vi "CreateHDF5NoDig.vi"() -> (0 "error out":errorcluster, 3 "File Handle":T1=16777216 format="%.0x")   [LabVIEW 2014]
uses:
  <vilib>/addons/h5labview2/base/hid_t.ctl
panel:
  in  "Material in Tank":string(combo)
  in  "Optional Comments":string
  in  "Run Type":string(combo)
  in  "Click OK when all data are entered.":bool
  in  "QDC Info, Ch0 - 7, left to right":T2={"Chanel Description"=["H0", "H1", "H2", "H3", "H4", "H5"], "Only Hodo?"=[TRUE, TRUE, TRUE, TRUE, TRUE, TRUE]}
  in  "Scaler Info":T2={"Chanel Description"=["H0", "H1", "H2", "H3", "H4", "H5", "CT", "M", "LED", "CT+M+LED", "S0", "S1", "S2", "S3", "S4", "S5", "S6", "S7"], "Only Hodo?"=[TRUE, TRUE, TRUE, TRUE, TRUE, TRUE, TRUE, TRUE, FALSE, FALSE, FALSE, FALSE, FALSE, FALSE, FALSE, FALSE, FALSE, FALSE]}
  in  "TDC Info":T2={"Chanel Description"=["H0", "H1", "H2", "H3", "H4", "H5", "CT", "M", "LED", "CT+M+LED", "S0", "S1", "S2", "S3", "S4", "S5", "S6", "S7"], "Only Hodo?"=[TRUE, TRUE, TRUE, TRUE, TRUE, TRUE, TRUE, FALSE, FALSE, FALSE, FALSE, FALSE, FALSE, FALSE, FALSE, FALSE, FALSE, FALSE]}
  in  "Trigger Bit Descriptions":string[](array[string])=["Cosmic Trigger (H0+H2)x(H1+H3)", "Multiplicity (S>1)", "LED pulse", "CT+M+LED"]
  in  "Thermocouple Location":string[](array[string])=["None", "None"]
  in  "HDF5 File Path":path=path "C:/Users/lbignell/Desktop/dummy3.h5" caption="HDF5 File Path (file name automatically generated)"
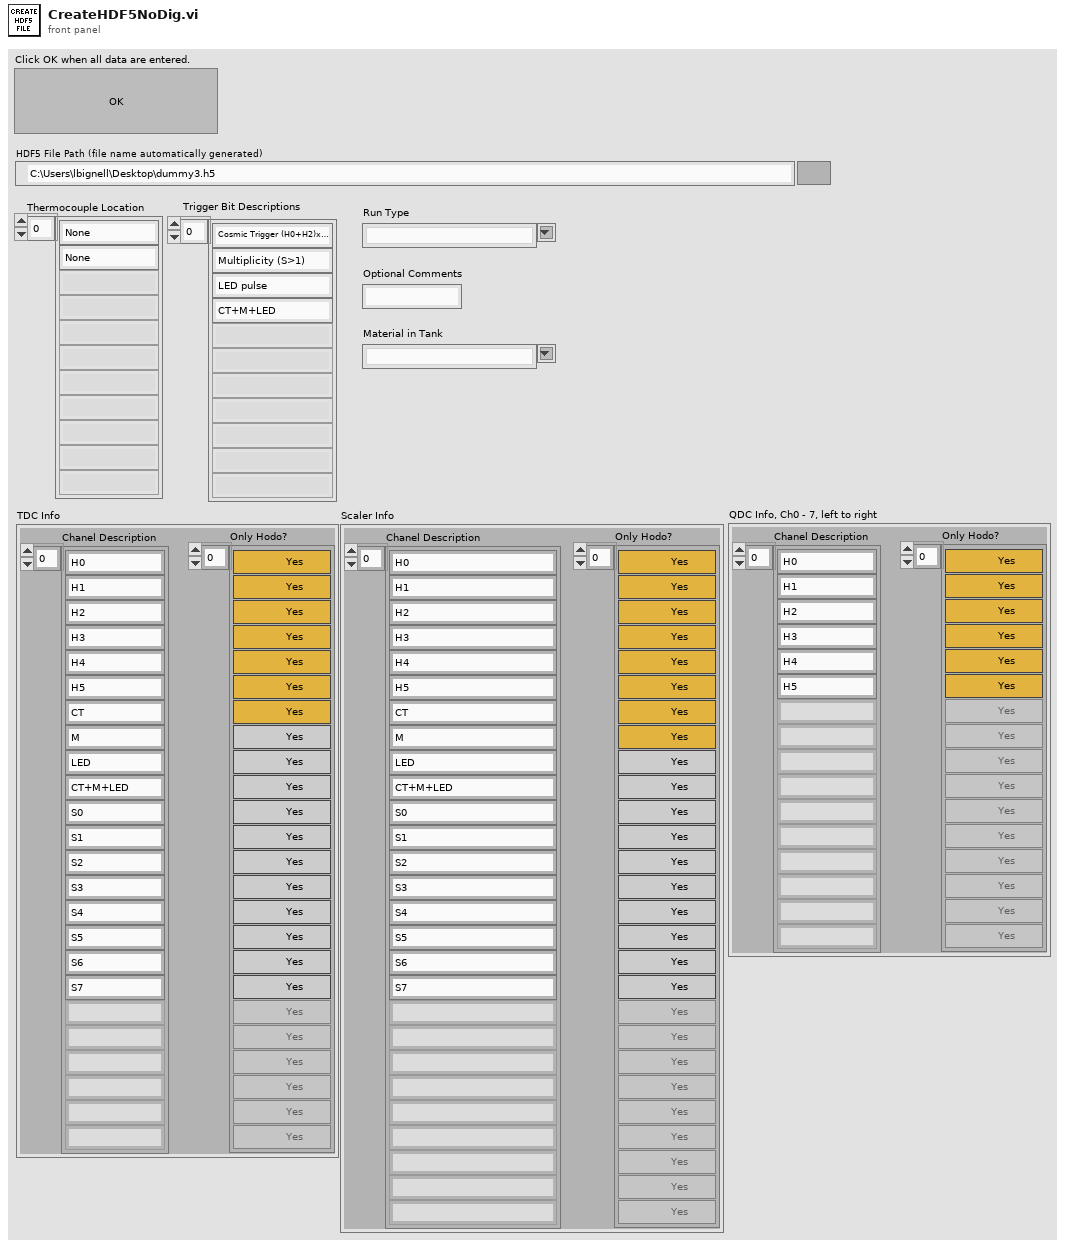
[diagram p1: front panel]
types:
  T1 = typedef "hid_t.ctl" = i32
  T2 = cluster{"Chanel Description":string[], "Only Hodo?":bool[]}
  T3 = cluster{"Module Description":string[], "Module Model":string[], "Module Address":u32[]}
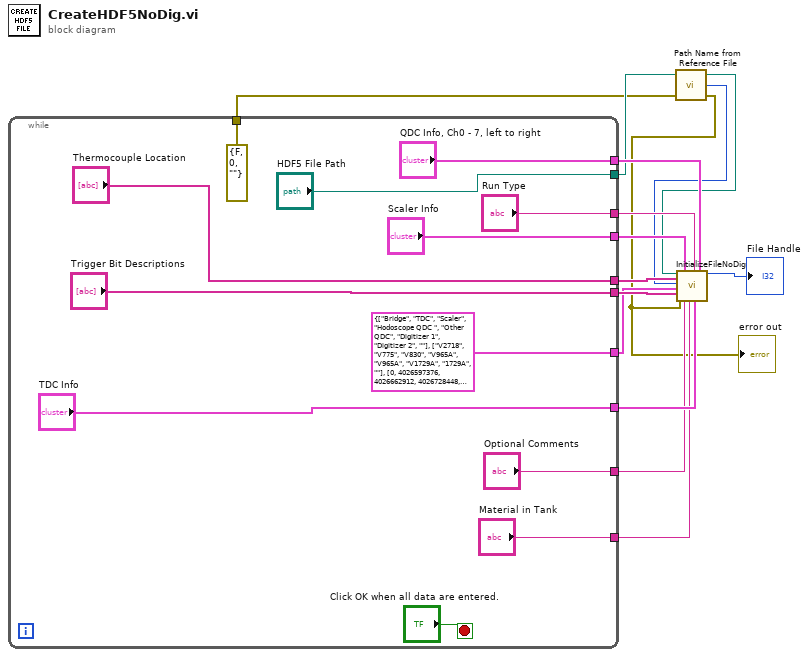
[diagram p0: block diagram]
diagram:
  n1 = while {
    tunnel: ["Thermocouple Location"] -> w15
    tunnel: ["Trigger Bit Descriptions"] -> w14
    tunnel: ["QDC Info, Ch0 - 7, left to right"] -> w13
    tunnel: ["Scaler Info"] -> w12
    tunnel: ["TDC Info"] -> w11
    tunnel: [T3 {"Module Description"=["Bridge", "TDC", "Scaler", "Hodoscope QDC ", "Other QDC", "Digitizer 1", "Digitizer 2", ""], "Module Model"=["V2718", "V775", "V830", "V965A", "V965A", "V1729A", "1729A", ""], "Module Address"=[0, 4026597376, 4026662912, 4026728448, 4026793984, 4026859520, 4026925056]} ("VME Configuration")] -> w9
    tunnel: ["Run Type"] -> w6
    tunnel: ["Optional Comments"] -> w7
    tunnel: ["Material in Tank"] -> w8
    tunnel: ["HDF5 File Path"] -> w5
    tunnel: [errorcluster {"status"=FALSE, "code"=0, "source"=""} ("error in")] -> w4
    stop <- "Click OK when all data are entered." stop-if-true
  }
  n2 = call "Path Name from Reference File"("error in"=w4, "Base Path"=w5) -> ("error out"=w3:errorcluster, "Run Number"=w2:i32, "Unique Path"=w1:path)  [unwired: 1 in]
  "error out" <- w3
  n3 = call "InitializeFileNoDig.vi"("File Path"=w1, "Thermocouple Location"=w15, "Run Number"=w2, "VME Configuration"=w9, "Trigger Bit Descriptions"=w14, "error in"=w3, "Scaler Info"=w12, "Optional Comments"=w7, "Material in Tank"=w8, "Run Type"=w6, "TDC Info"=w11, "QDC Info"=w13) -> ("File Handle"=→"File Handle":T1)  [unwired: 6 in, 1 out]
